vi "STAGE+mono+counter_edit4.vi"() -> ()   [LabVIEW 2017]
panel:
  out "XY Graph":cluster{"Y":dbl[], "Y":dbl[]}[](graph)
  in  "Integrating time, 10^-7 sec":dbl=10000000.0
  out "Timeout 2":bool
  in  "scan from":i32=2600
  in  "scan to":i32=4000
  in  "?":bool
  in  "Exit Labview":bool
  in  "step size":dbl=10.0 min=0.0
  in  "?":bool
  out "Spectrum":waveform(dbl)(graph)
  out "Counts":i32
  in  "value (0)":dbl=-9.0
  out "Current WL Wavelength  2":u16 caption="Current Wavelength"
  out "Grt# 2":u8=1 min=1 max=3 step=1
  out "Blaze (nm)":u32=300
  out "Groove/mm":u32=1200
  in  "?":bool
  in  "Channel B Input":u16(ring)=2 items=["Input 1"=1, "Input 2"=2]
  in  "Trigger mode":u16(ring) items=["10 MHz"=0, "Input 2"=2, "Input T"=3]
  out "Current WL Wavelength":u16 caption="Current Wavelength"
  in  "Integrating time, 10^-7 sec":dbl=10000000.0
  in  "gate A mode (CW:0)":i16(slide) scale=0.0..2.0 scale format="%.2f"
  in  "Channel A Input":u16(ring)=1 items=["10 MHz", "Input 1"]
  in  "Time between measurements\n at one point (s)/Dwell Time":dbl=0.002 min=0.002 max=60.0 step=0.001
  in  "Number of Measurements\n to take at one point/ Number of Periods":u16=1 min=1 max=2000 step=1
  in  "Count Mode":u16(ring) items=["A,B for Preset T", "A-B for Preset T", "A+B for Preset T", "A for Preset B"]
  in  "GPIB address":string="23"
  out "Timeout":bool
  out "Serial":u32=12345
  out "Grt#":u8=1 min=1 max=3 step=1
  out "Blaze (nm)":u32=300
  out "Groove/mm":u32=1200
  out "time delay":u32=450000 min=1
  out "Mono port":T1(ring)
  in  "Get position":bool
  out "Position status":dbl format="%.3f"
  in  "Target position":dbl format="%.3f"
  in  "Move":bool
  in  "Motor OFF":bool
  in  "Motor ON":bool
  in  "Step Size [um]":i32=10
  in  "Axis":i32=1
  in  "Rep Rate [Hz]":dbl=500.0
  out "Shots":dbl
  in  "Averaging Time [s]":dbl=0.1
  out "Current Point":i32
  out "Slide":i32(slide) scale=0.0..100.0
  out "Current Position [mm]":dbl
  in  "Axis initial position [mm]":dbl
  out "Axis final Position [mm]":dbl
  in  "Data Points (100 default)":i32=100
  in  "Collect Data!":bool
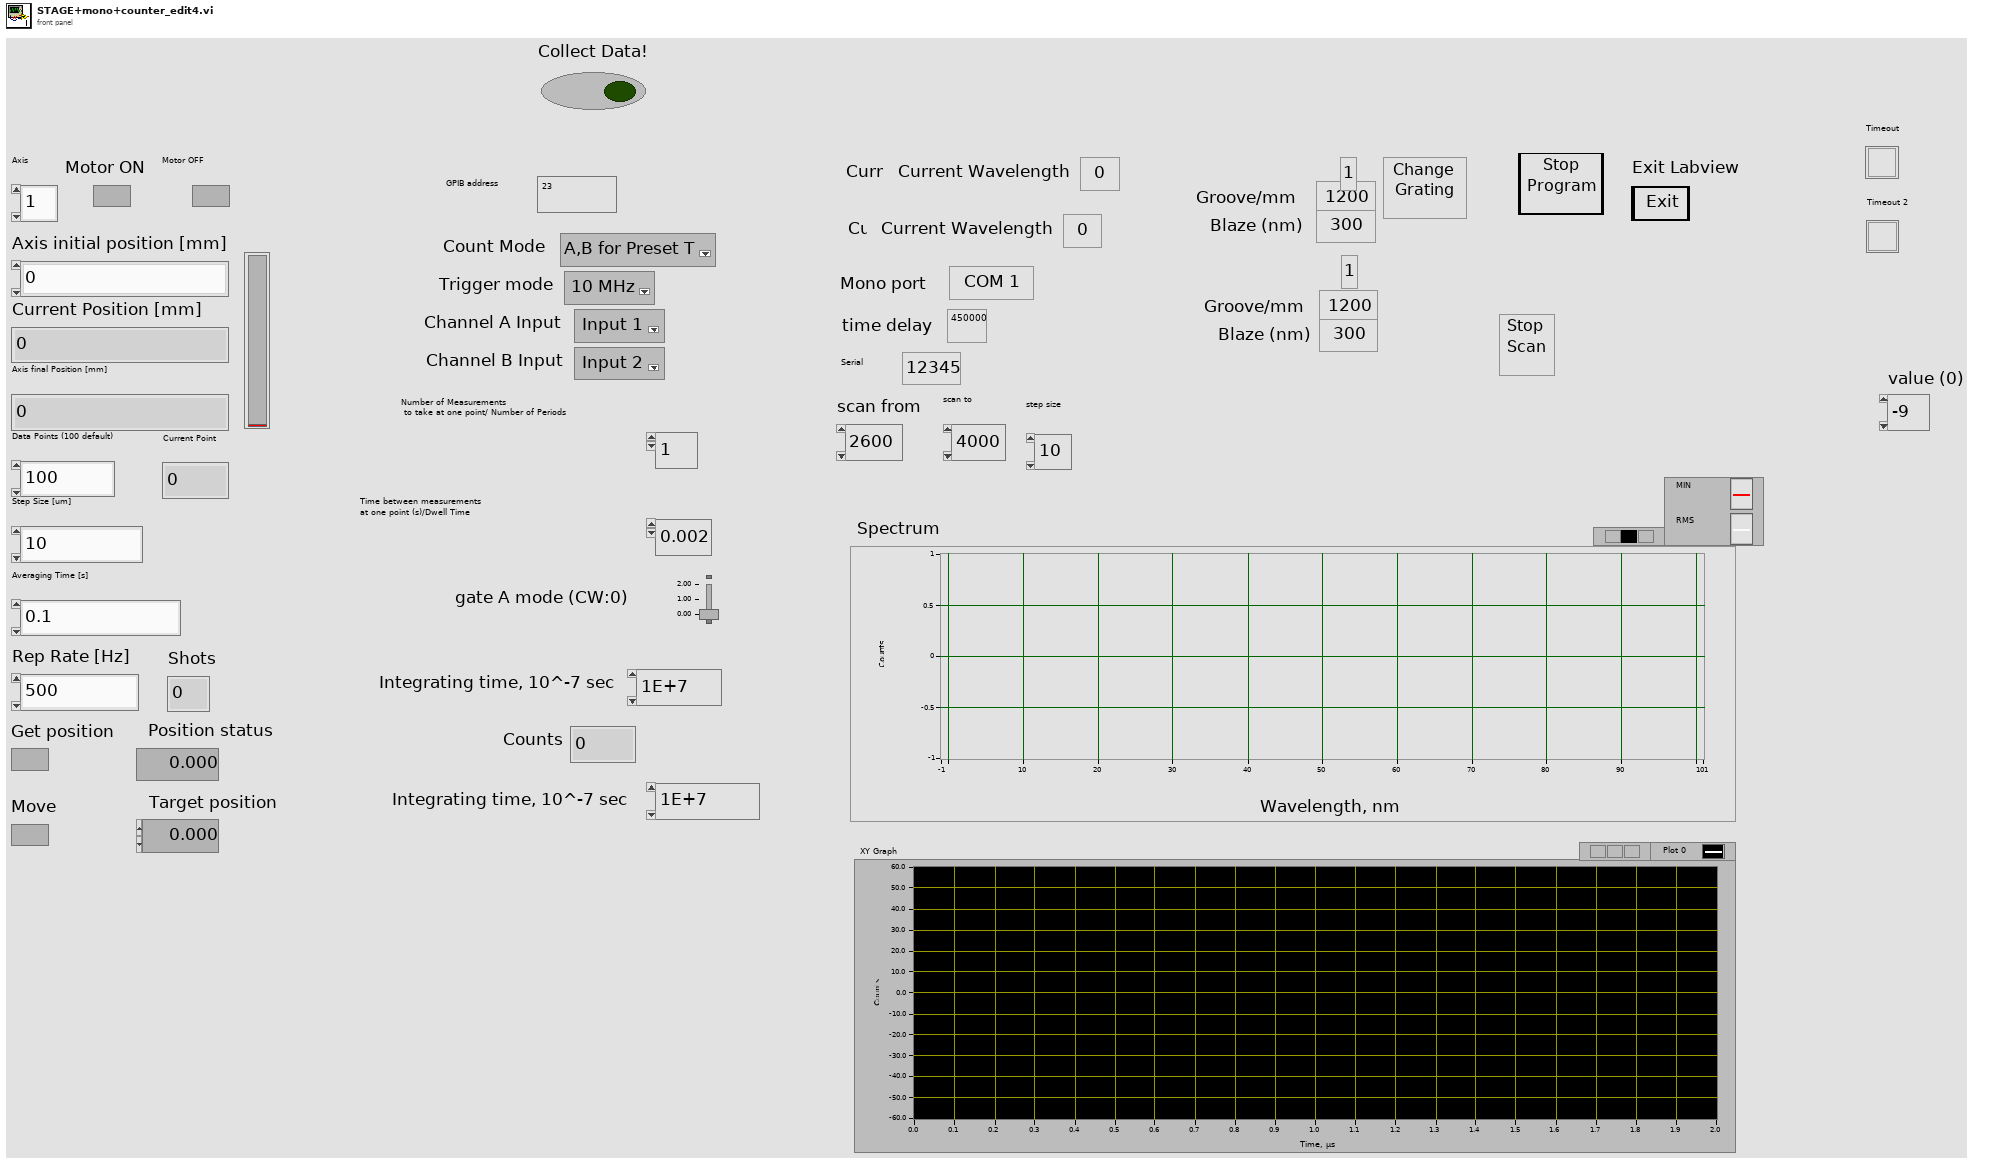
[diagram p1: front panel]
types:
  T1 = enum8{"COM 1", "COM 2", "COM 3", "COM 4", "COM 5", "COM 6", "COM 7", "COM 8", "COM 9"}
  T2 = cluster{"input XON/XOFF":bool, "input HW Handshake":bool, "input alt HW HShk":bool, "output XON/XOFF":bool, "output HW Handshake":bool, "output alt HW HShk":bool, "XOFF byte":u8, "XON byte":u8, "parity error byte":u16}
  T3 = enum16{"no parity", "odd parity", "even parity", "mark parity", "space parity"}
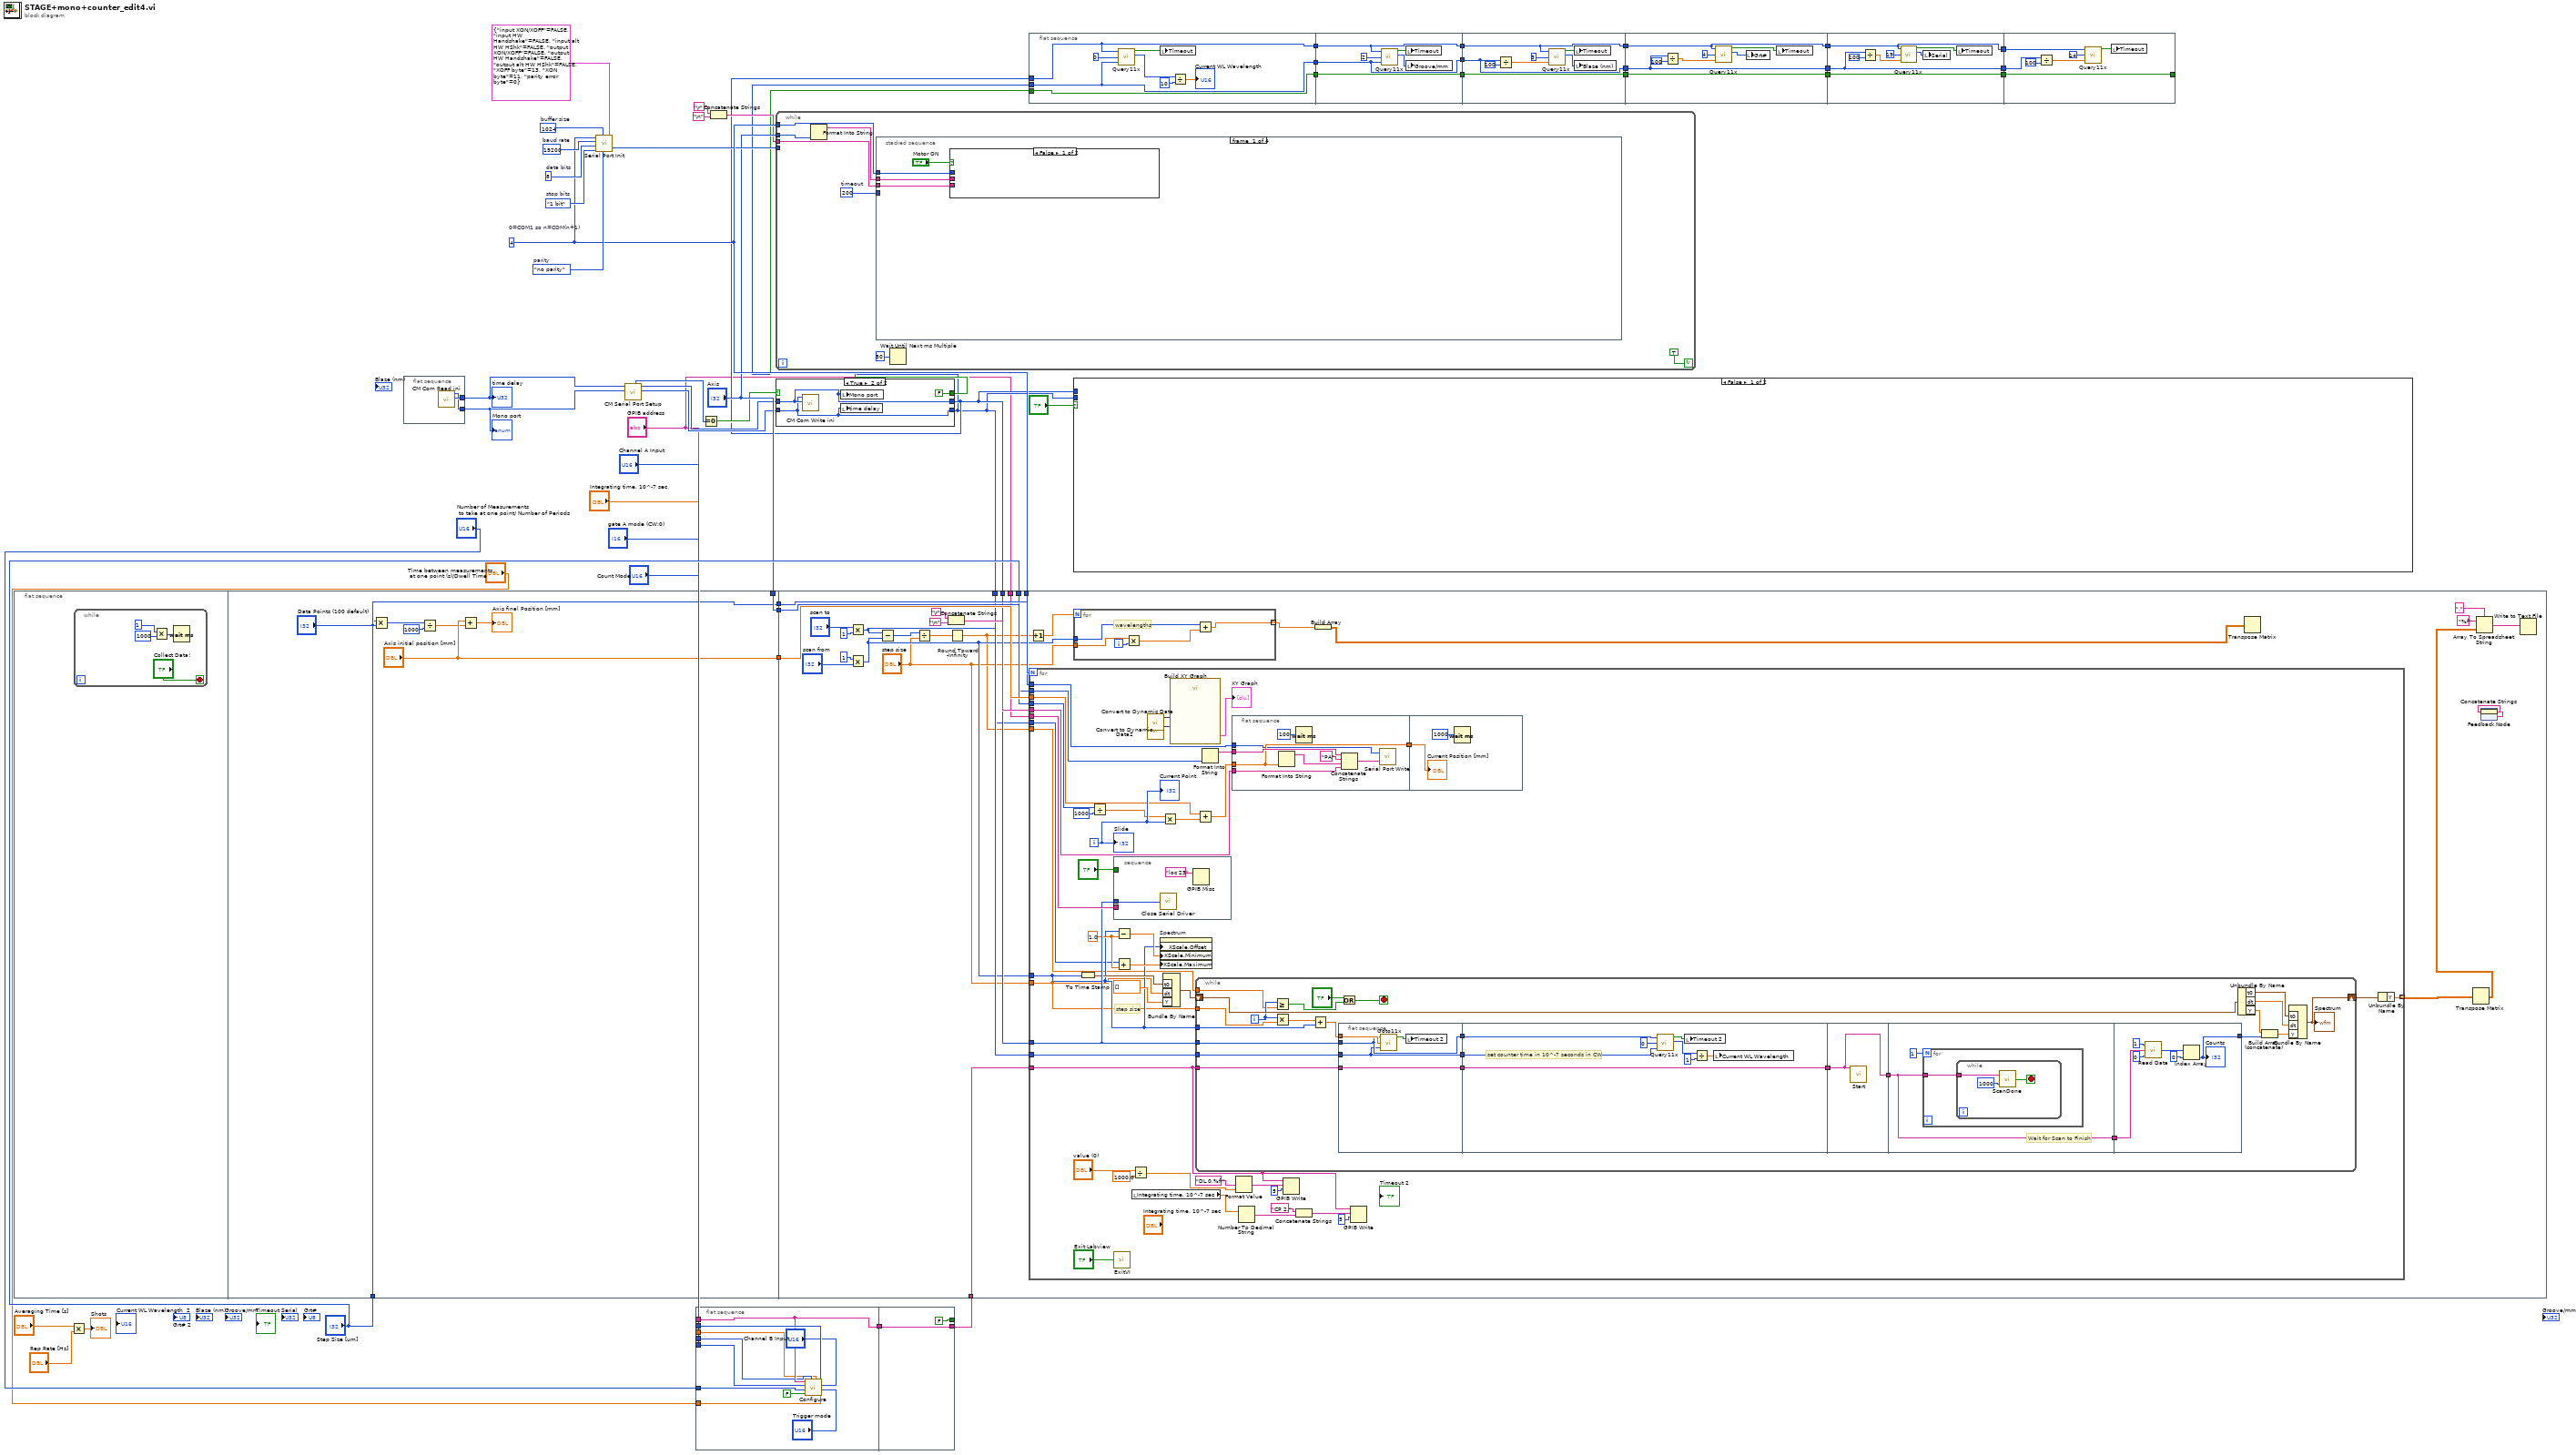
[diagram p0: block diagram]
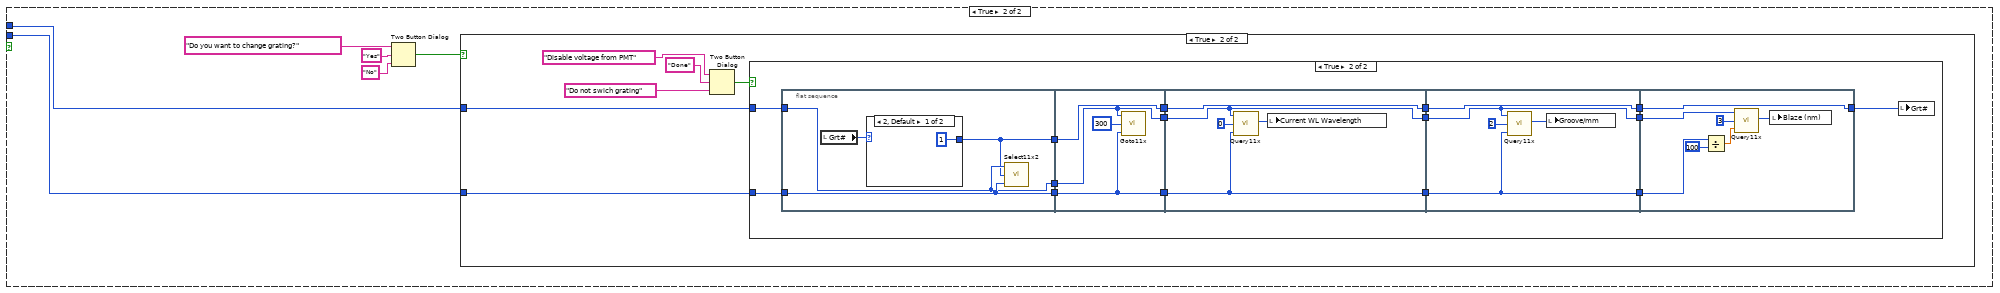
[diagram p2: hidden frame]
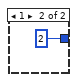
[diagram p5: hidden frame]
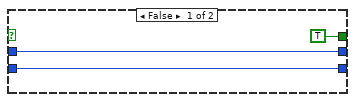
[diagram p6: hidden frame]
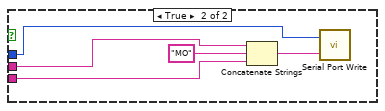
[diagram p7: hidden frame]
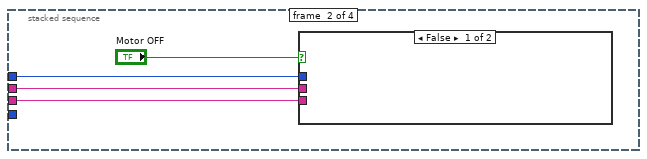
[diagram p8: hidden frame]
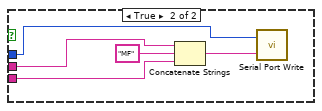
[diagram p9: hidden frame]
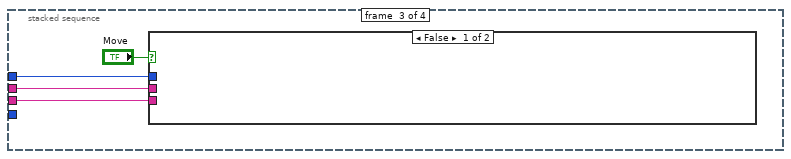
[diagram p10: hidden frame]
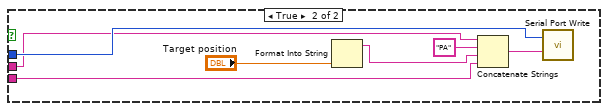
[diagram p11: hidden frame]
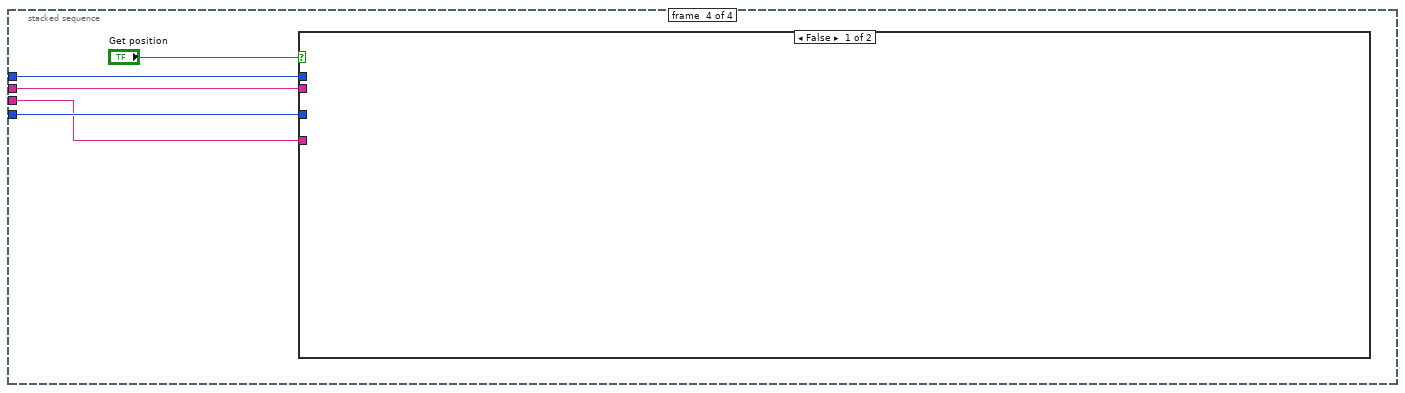
[diagram p12: hidden frame]
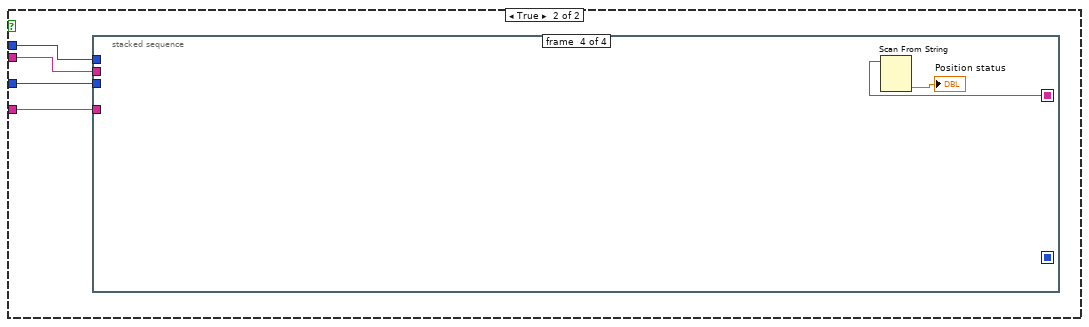
[diagram p13: hidden frame]
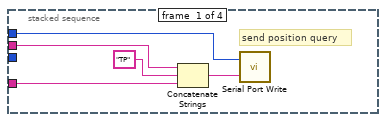
[diagram p14: hidden frame]
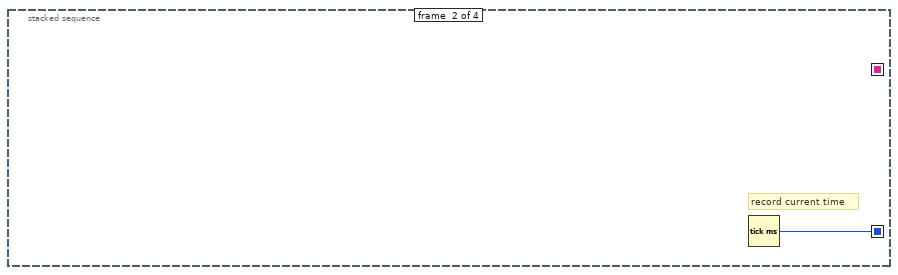
[diagram p15: hidden frame]
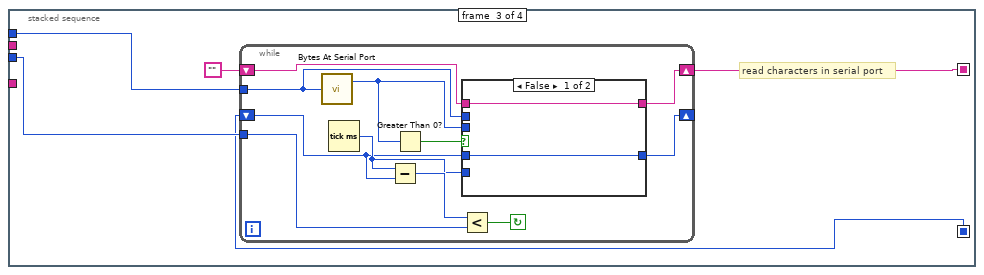
[diagram p16: hidden frame]
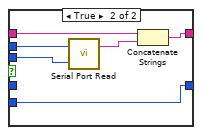
[diagram p17: hidden frame]
diagram:
  w43 = u32 19200  # baud rate
  w42 = u16 8  # data bits
  w41 = enum16{"1 bit", "1.5 bits", "2 bits"}."1 bit"  # stop bits
  w46 = T3."no parity"  # parity
  w40 = 4  # 0=COM1 so n=COM(n+1)
  w45 = u16 1024  # buffer size
  n1 = flat-sequence {
    tunnel: ["Data Points (100 default)"] -> w53
    tunnel: "Axis" -> [w65]
    tunnel: ["Axis initial position [mm]"] -> w52
    tunnel: "Step Size [um]" -> [w58]
    tunnel: [w65] -> w51
    tunnel: w53 -> [w97]
    tunnel: w52 -> [w96]
    tunnel: "Step Size [um]" -> [w95]
    tunnel: w51 -> [w94]
    tunnel: w40 -> [w90]
    tunnel: w4 -> [w89]
    tunnel: w3 -> [w88]
    tunnel: w2 -> [w87]
    tunnel: "GPIB address" -> [w86]
    frame #0 {
      n2 = while {
        stop <- "Collect Data!" stop-if-true
        n3 = Multiply(x=1, y=1000) -> (x*y=w57:i32)
        n4 = Wait (ms)(milliseconds to wait=w57) -> ()  [unwired: 1 out]
      }
    }
    frame #1 {
      n5 = Multiply(x=w58, y="Data Points (100 default)") -> (x*y=w61:i32)
      n6 = Divide(x=w61, y=1000) -> (x/y=w60:dbl)
      n7 = Add(x="Axis initial position [mm]", y=w60) -> (x+y=→"Axis final Position [mm]":dbl)
    }
    frame #2 {
      n8 = Multiply(x="scan to", y=1) -> (x*y=w78:i32)
      n9 = Multiply(x=1, y="scan from") -> (x*y=w81:i32)
      n10 = Subtract(x=w78, y=w81) -> (x-y=w76:i32)
      n11 = Divide(x=w76, y="step size") -> (x/y=w75:dbl)
      n12 = Concatenate Strings("\r", "\n") -> (w91:string)
      n13 = Round Toward -Infinity(1:w75) -> (0:w74:dbl)
      n14 = for {
        N: w97 -> [_]
        tunnel: w96 -> [w145]
        tunnel: w95 -> [w141]
        tunnel: w94 -> [w138]
        tunnel: w91 -> [w135]
        tunnel: w90 -> [w136]
        tunnel: w89 -> [w133]
        tunnel: w88 -> [w130]
        tunnel: w87 -> [w132]
        tunnel: w86 -> [w131]
        tunnel: [w103] -> w67 mode=indexing
        tunnel: w81 -> [w107]
        tunnel: w78 -> [w106]
        tunnel: "step size" -> [w105]
        tunnel: w74 -> [w104]
        i -> [w146]
        w127 = 1.0 ("x")
        # "step size"
        n15 = To Time Stamp(1:w107) -> (0:w123:timestamp)
        n16 = Divide(x=w141, y=1000) -> (x/y=w140:dbl)
        n17 = stacked-sequence {
          tunnel: "?" -> [_]
          tunnel: w130 -> [w199]
          tunnel: w131 -> [_]
          frame #0 {
            n18 = call <vilib>:"Close Serial Driver.vi"("port number"=w199) -> ()  [unwired: 1 out]
            n19 = GPIB Misc(0:"loc 23" ("command string")) -> ()  [unwired: 1 in, 3 out]
          }
        }
        n20 = call "ExitVI.vi"("Exit Labview"="Exit Labview") -> ()
        n21 = Subtract(x=w107, y=w127) -> (x-y=w126:dbl)
        n22 = Add(x=w106, y=w127) -> (x+y=w128:dbl)
        n23 = local read "Integrating time, 10^-7 sec"() -> (w125:dbl)
        n24 = Divide(x="value (0)", y=1000.0) -> (x/y=w111:dbl)
        n25 = call "Convert to Dynamic Data"() -> ("Dynamic Data Type"=w108:dynamicdata)  [unwired: 4 in]
        n26 = call "Convert to Dynamic Data2"() -> ("Dynamic Data Type"=w109:dynamicdata)  [unwired: 4 in]
        n27 = property on="Spectrum" class="WFGraph (strict)"("XScale.Offset"=w107, "XScale.Minimum"=w126, "XScale.Maximum"=w128) -> ()  [unwired: 2 in, 2 out]
        n28 = Multiply(x=w140, y=w146) -> (x*y=w144:dbl)
        n29 = Bundle By Name("t0"=w123, "dt"=w105, "Y"=dbl[] []) -> (w122:waveform(dbl))  [unwired: 1 in]
        n30 = call "Build XY Graph"("Y Input"=w109, "X Input"=w108) -> ("XY Graph"=→"XY Graph":cluster{"Y":dbl[], "Y":dbl[]}[])  [unwired: 3 in, 6 out]
        n31 = while {
          tunnel: w130 -> [w170]
          tunnel: w132 -> [w169]
          shift-right: [w159] -> w117
          shift-left: w122 -> [w167]
          tunnel: w133 -> [w158]
          tunnel: w107 -> [w149]
          tunnel: w105 -> [w148]
          tunnel: w104 -> [w147]
          i -> [w164]
          stop <- w168 stop-if-true
          n32 = Greater Or Equal?(x=w164, y=w147) -> (x >= y?=w160:bool)
          n33 = Multiply(x=w164, y=w148) -> (x*y=w171:dbl)
          n34 = Add(x=w171, y=w149) -> (x+y=w150:dbl)
          n35 = flat-sequence {
            tunnel: w150 -> [w176]
            tunnel: w170 -> [w175]
            tunnel: [w175] -> w156
            tunnel: w169 -> [w174]
            tunnel: [w174] -> w155
            tunnel: w158 -> [w172]
            tunnel: [w172] -> w154
            tunnel: w156 -> [w183]
            tunnel: w155 -> [w182]
            tunnel: w154 -> [w180]
            tunnel: [w180] -> w153
            tunnel: w153 -> [w185]
            tunnel: [w185] -> w152
            tunnel: w152 -> [w186]
            tunnel: [w186] -> w151
            tunnel: w151 -> [w193]
            tunnel: [w192] -> w157
            frame #0 {
              n36 = call "Goto11x.vi"("time delay"=w174, "WAVELENGTH"=w176, "port number"=w175) -> ("timeout"=w173:bool)  [unwired: 2 out]
              n37 = local write "Timeout 2"(w173) -> ()
            }
            frame #1 {
              # "set counter time in 10^-7 seconds in CW"
              n38 = call "Query11x.vi"("port number"=w183, "QUERY"=0, "time delay"=w182) -> ("timeout"=w181:bool, "STATUS MESSAGE"=w179:u16)  [unwired: 2 out]
              n39 = local write "Timeout 2"(w181) -> ()
              n40 = Divide(x=w179, y=1) -> (x/y=w178:dbl)
              n41 = local write "Current WL Wavelength"(w178) -> ()
            }
            frame #2 {
              n42 = call "Start.vi"("GPIB Address"=w185) -> ()  [unwired: 9 in]
            }
            frame #3 {
              # "Wait for Scan to Finish"
              n43 = for {
                N: 1 -> [_]
                tunnel: w186 -> [w188]
                n44 = while {
                  tunnel: w188 -> [w189]
                  stop <- w191 stop-if-true
                  n45 = call "ScanDone.vi"("Wait (ms)"=1000, "GPIB Address"=w189) -> ("Scan Finished?"=w191:bool)
                }
              }
            }
            frame #4 {
              n46 = call "Read Data.vi"("Channel Number"=0, "GPIB Address"=w193, "Number of Datapoints"=1) -> ("Data"=w194:i32[])
              n47 = Index Array(array=w194, index=0) -> (element=w192:i32)
              "Counts" <- w192
            }
          }
          n48 = Or(x="?", y=w160) -> (x .or. y?=w168:bool)
          n49 = Unbundle By Name(w167) -> ("t0"=w165:timestamp, "dt"=w166:dbl, "Y"=w163:dbl[])
          n50 = Build Array (concatenate)(w163, w157) -> (w162:dbl[])
          n51 = Bundle By Name("t0"=w165, "dt"=w166, "Y"=w162) -> (w159:waveform(dbl))  [unwired: 1 in]
          "Spectrum" <- w159
        }
        n52 = Add(x=w145, y=w144) -> (x+y=w143:dbl)
        n53 = Format Into String(w138) -> (resulting string=w137:string)  [unwired: 3 in, 1 out]
        n54 = flat-sequence {
          tunnel: w143 -> [w202]
          tunnel: [w202] -> w139
          tunnel: w135 -> [w204]
          tunnel: w137 -> [w203]
          tunnel: w136 -> [w200]
          tunnel: w139 -> [w208]
          frame #0 {
            n55 = Format Into String(w202) -> (resulting string=w201:string)  [unwired: 3 in, 1 out]
            n56 = Wait (ms)(milliseconds to wait=u32 100) -> ()  [unwired: 1 out]
            n57 = Concatenate Strings(w203, "PA" ("Substring"), w201, w204) -> (w206:string)
            n58 = call <vilib>:"Serial Port Write.vi"("string to write"=w206, "port number"=w200) -> ()  [unwired: 1 out]
          }
          frame #1 {
            n59 = Wait (ms)(milliseconds to wait=u32 1000) -> ()  [unwired: 1 out]
            "Current Position [mm]" <- w208
          }
        }
        n60 = Format Value(format string="DL 0,%f;", value (0)=w111) -> (output string=w115:string)  [unwired: 1 in]
        n61 = Number To Decimal String(number=w125) -> (decimal integer string=w120:string)  [unwired: 1 in]
        n62 = GPIB Write(0:w133, 1:w115, 2:i16 5 ("mode (0)")) -> ()  [unwired: 2 in, 2 out]
        n63 = Concatenate Strings("CP 2,", w120) -> (w118:string)
        n64 = GPIB Write(0:w133, 1:w118, 2:i16 5 ("mode (0)")) -> ()  [unwired: 2 in, 2 out]
        n65 = Unbundle By Name(w117) -> ("Y"=w103:dbl[])
        "Current Point" <- w146
        "Slide" <- w146
      }
      n66 = Increment(x=w74) -> (x+1=w73:dbl)
      n67 = for {
        N: w73 -> [_]
        tunnel: "step size" -> [w102]
        tunnel: w81 -> [w100]
        tunnel: [w98] -> w71 mode=indexing
        i -> [w101]
        # "wavelengths"
        n68 = Multiply(x=w102, y=w101) -> (x*y=w99:dbl)
        n69 = Add(x=w100, y=w99) -> (x+y=w98:dbl)
      }
      n70 = Build Array(w71) -> (w68:dbl[][])
      n71 = Transpose Matrix(1:w68) -> ()  [unwired: 1 out]
      n72 = Transpose Matrix(1:w67) -> (0:w66:dbl[][])
      n73 = Array To Spreadsheet String(delimiter (Tab)=",", array=w66, 3:"%f" ("format string")) -> (spreadsheet string=w72:string)
      n74 = feedback #1() -> (w69:string)  [unwired: 1 in]
      n75 = Concatenate Strings(w69) -> (w70:string)
      n76 = feedback-in #1(w70) -> ()
      n77 = Write to Text File(text=w72) -> ()  [unwired: 3 in, 3 out]
    }
  }
  n78 = Multiply(x="Averaging Time [s]", y="Rep Rate [Hz]") -> (x*y=→"Shots":dbl)
  n79 = flat-sequence {
    tunnel: [w211] -> w18
    tunnel: [w210] -> w17
    frame #0 {
      n80 = call "CM Com Read ini.vi"() -> ("Mono port"=w210:T1, "time delay1"=w211:u32)  [unwired: 7 in]
    }
  }
  n81 = call <vilib>:"Serial Port Init.vi"("flow control etc."=T2 {"input XON/XOFF"=FALSE, "input HW Handshake"=FALSE, "input alt HW HShk"=FALSE, "output XON/XOFF"=FALSE, "output HW Handshake"=FALSE, "output alt HW HShk"=FALSE, "XOFF byte"=13, "XON byte"=11, "parity error byte"=0}, "parity"=w46, "buffer size"=w45, "stop bits"=w41, "data bits"=w42, "baud rate"=w43, "port number"=w40) -> ("error code"=w39:i32)
  n82 = call "CM Serial Port Setup.vi"("COM port"=w17, "time delay"=w18) -> ("time delay1"=w13:u32, "DK port Out"=w14:T1, "error code"=w16:i32)  [unwired: 7 in]
  n83 = flat-sequence {
    tunnel: "GPIB address" -> [w219]
    tunnel: [w219] -> w19
    tunnel: "Count Mode" -> [w220]
    tunnel: "Number of Measurements\n to take at one point/ Number of Periods" -> [w217]
    tunnel: "Time between measurements\n at one point (s)/Dwell Time" -> [w216]
    tunnel: "Channel A Input" -> [w221]
    tunnel: "gate A mode (CW:0)" -> [w213]
    tunnel: "Integrating time, 10^-7 sec" -> [w212]
    tunnel: w19 -> [w222]
    tunnel: [w222] -> w4
    tunnel: [FALSE] -> _
    frame #0 {
      n84 = call "Configure.vi"("Dwell Time (s)"=w216, "Channel T Input"="Trigger mode", "Channel B Input"="Channel B Input", "Channel A Input"=w221, "Integrating time, 10^-7 sec"=w212, "gate mode (CW:0)"=w213, "Scan End Mode"=FALSE, "Number of Periods"=w217, "Count Mode"=w220, "GPIB Address"=w219) -> ()
    }
    frame #1 {
    }
  }
  n85 = Equal To 0?(x=w16) -> (x = 0?=w15:bool)
  n86 = Concatenate Strings("\r", "\n") -> (w35:string)
  n87 = while {
    tunnel: w40 -> [w226]
    tunnel: w35 -> [w227]
    tunnel: w39 -> [_]
    tunnel: "Axis" -> [w224]
    stop <- TRUE continue-if-true
    w225 = u32 200  # timeout
    n88 = Format Into String(w224) -> (resulting string=w228:string)  [unwired: 3 in, 1 out]
    n89 = stacked-sequence {
      tunnel: w228 -> [w232 w242 w251 w263]
      tunnel: w227 -> [w231 w241 w250 w260]
      tunnel: w226 -> [w233 w243 w252 w262]
      tunnel: w225 -> [_ _ _ w261]
      frame #0 {
        n90 = case shown="False" "Motor ON" {
          tunnel: w233 -> [_ w239]
          tunnel: w232 -> [_ w236]
          tunnel: w231 -> [_ w235]
          frame False {
          }
          frame True {
            n91 = Concatenate Strings(w236, "MO" ("Substring"), w235) -> (w237:string)
            n92 = call <vilib>:"Serial Port Write.vi"("string to write"=w237, "port number"=w239) -> ()  [unwired: 1 out]
          }
        }
      }
      frame #1 {
        n93 = case shown="False" "Motor OFF" {
          tunnel: w243 -> [_ w248]
          tunnel: w242 -> [_ w245]
          tunnel: w241 -> [_ w244]
          frame False {
          }
          frame True {
            n94 = Concatenate Strings(w245, "MF" ("Substring"), w244) -> (w246:string)
            n95 = call <vilib>:"Serial Port Write.vi"("string to write"=w246, "port number"=w248) -> ()  [unwired: 1 out]
          }
        }
      }
      frame #2 {
        n96 = case shown="False" "Move" {
          tunnel: w252 -> [_ w259]
          tunnel: w251 -> [_ w256]
          tunnel: w250 -> [_ w255]
          frame False {
          }
          frame True {
            n97 = Format Into String("Target position") -> (resulting string=w253:string)  [unwired: 3 in, 1 out]
            n98 = Concatenate Strings(w256, "PA" ("Substring"), w253, w255) -> (w257:string)
            n99 = call <vilib>:"Serial Port Write.vi"("string to write"=w257, "port number"=w259) -> ()  [unwired: 1 out]
          }
        }
      }
      frame #3 {
        n100 = case shown="False" "Get position" {
          tunnel: w263 -> [_ w268]
          tunnel: w262 -> [_ w267]
          tunnel: w261 -> [_ w266]
          tunnel: w260 -> [_ w265]
          frame False {
          }
          frame True {
            n101 = stacked-sequence {
              seq-local: [_ w274 _ _] -> [_ _ w276 _]
              seq-local: [_ _ w275 _] -> [_ _ _ w300]
              tunnel: w268 -> [w271 _ _ _]
              tunnel: w267 -> [w270 _ w279 _]
              tunnel: w266 -> [_ _ w277 _]
              tunnel: w265 -> [w269 _ _ _]
              frame #0 {
                # "send position query"
                n102 = Concatenate Strings(w271, "TP" ("Substring"), w269) -> (w272:string)
                n103 = call <vilib>:"Serial Port Write.vi"("string to write"=w272, "port number"=w270) -> ()  [unwired: 1 out]
              }
              frame #1 {
                # "record current time"
                n104 = Tick Count (ms)() -> (millisecond timer value=w274:u32)
              }
              frame #2 {
                # "read characters in serial port"
                n105 = while {
                  shift-left: w276 -> [w280]
                  shift-right: [w281] -> _
                  tunnel: w277 -> [w284]
                  shift-left: "" -> [w287]
                  shift-right: [w286] -> w275
                  tunnel: w279 -> [w288]
                  stop <- w283 continue-if-true
                  n106 = call <vilib>:"Bytes At Serial Port.vi"("port number"=w288) -> ("byte count"=w289:u32)  [unwired: 1 out]
                  n107 = Tick Count (ms)() -> (millisecond timer value=w282:u32)
                  n108 = Subtract(x=w282, y=w280) -> (x-y=w285:u32)
                  n109 = Greater Than 0?(x=w289) -> (x > 0?=w290:bool)
                  n110 = case shown="False" w290 {
                    tunnel: w289 -> [_ w298]
                    tunnel: w288 -> [_ w297]
                    tunnel: w287 -> [w292 w295]
                    tunnel: [w292 w294] -> w286
                    tunnel: [w291 w293] -> w281
                    tunnel: w282 -> [_ w293]
                    tunnel: w280 -> [w291 _]
                    frame False {
                    }
                    frame True {
                      n111 = call <vilib>:"Serial Port Read.vi"("requested byte count"=w298, "port number"=w297) -> ("string read"=w296:string)  [unwired: 1 out]
                      n112 = Concatenate Strings(w295, w296) -> (w294:string)
                    }
                  }
                  n113 = Less?(x=w285, y=w284) -> (x < y?=w283:bool)
                }
              }
              frame #3 {
                n114 = Scan From String(input string=w300) -> (output 1=→"Position status":dbl)  [unwired: 4 in, 3 out]
              }
            }
          }
        }
      }
    }
    n115 = Wait Until Next ms Multiple(millisecond multiple=u32 50) -> ()  [unwired: 1 out]
  }
  n116 = case shown="True" w15 {
    tunnel: w14 -> [w303 w306]
    tunnel: w13 -> [w302 w305]
    tunnel: [w303 w306] -> w3
    tunnel: [w302 w305] -> w2
    tunnel: [TRUE FALSE] -> w12
    frame False {
    }
    frame True {
      n117 = call "CM Com Write ini.vi"("time delay1"=w306, "Mono port"=w305) -> ()  [unwired: 7 in]
      n118 = local write "Mono port"(w306) -> ()
      n119 = local write "time delay"(w305) -> ()
    }
  }
  n120 = flat-sequence {
    tunnel: w2 -> [w312]
    tunnel: [w312] -> w34
    tunnel: w3 -> [w314]
    tunnel: [w314] -> w33
    tunnel: w12 -> [w310]
    tunnel: [w310] -> w32
    tunnel: w34 -> [w317]
    tunnel: [w317] -> w31
    tunnel: w33 -> [w319]
    tunnel: [w319] -> w30
    tunnel: w32 -> [w315]
    tunnel: [w315] -> w29
    tunnel: w31 -> [w327]
    tunnel: [w327] -> w28
    tunnel: w30 -> [w324]
    tunnel: [w324] -> w27
    tunnel: w29 -> [w321]
    tunnel: [w321] -> w26
    tunnel: w28 -> [w335]
    tunnel: [w335] -> w25
    tunnel: w27 -> [w332]
    tunnel: [w332] -> w24
    tunnel: w26 -> [w329]
    tunnel: [w329] -> w23
    tunnel: w25 -> [w343]
    tunnel: [w343] -> w22
    tunnel: w24 -> [w340]
    tunnel: [w340] -> w21
    tunnel: w23 -> [w337]
    tunnel: [w337] -> w20
    tunnel: w22 -> [w350]
    tunnel: w21 -> [w347]
    tunnel: [w345] -> _
    tunnel: w20 -> [w345]
    frame #0 {
      n121 = call "Query11x.vi"("port number"=w314, "QUERY"=u16 0, "time delay"=w312) -> ("timeout"=w311:bool, "STATUS MESSAGE"=w309:u16)  [unwired: 2 out]
      n122 = local write "Timeout"(w311) -> ()
      n123 = Divide(x=w309, y=10 ("Numeric")) -> (x/y=→"Current WL Wavelength":dbl)
    }
    frame #1 {
      n124 = call "Query11x.vi"("port number"=w319, "QUERY"=u16 2, "time delay"=w317) -> ("timeout"=w316:bool, "STATUS MESSAGE"=w318:u16)  [unwired: 2 out]
      n125 = local write "Timeout"(w316) -> ()
      n126 = local write "Groove/mm"(w318) -> ()
    }
    frame #2 {
      n127 = Divide(x=w327, y=i16 100 ("device (1)")) -> (x/y=w325:dbl)
      n128 = call "Query11x.vi"("port number"=w324, "QUERY"=u16 3, "time delay"=w325) -> ("timeout"=w322:bool, "STATUS MESSAGE"=w323:u16)  [unwired: 2 out]
      n129 = local write "Timeout"(w322) -> ()
      n130 = local write "Blaze (nm)"(w323) -> ()
    }
    frame #3 {
      n131 = Divide(x=w335, y=i16 100 ("device (1)")) -> (x/y=w333:dbl)
      n132 = call "Query11x.vi"("port number"=w332, "QUERY"=u16 4, "time delay"=w333) -> ("timeout"=w330:bool, "STATUS MESSAGE"=w331:u16)  [unwired: 2 out]
      n133 = local write "Grt#"(w331) -> ()
      n134 = local write "Timeout"(w330) -> ()
    }
    frame #4 {
      n135 = Divide(x=w343, y=i16 100 ("device (1)")) -> (x/y=w341:dbl)
      n136 = call "Query11x.vi"("port number"=w340, "QUERY"=u16 19, "time delay"=w341) -> ("timeout"=w338:bool, "STATUS MESSAGE"=w339:u16)  [unwired: 2 out]
      n137 = local write "Serial"(w339) -> ()
      n138 = local write "Timeout"(w338) -> ()
    }
    frame #5 {
      n139 = Divide(x=w350, y=i16 100 ("device (1)")) -> (x/y=w348:dbl)
      n140 = call "Query11x.vi"("port number"=w347, "QUERY"=u16 14, "time delay"=w348) -> ("timeout"=w346:bool)  [unwired: 3 out]
      n141 = local write "Timeout"(w346) -> ()
    }
  }
  n142 = case shown="False" "?" {
    tunnel: w2 -> [_ w353]
    tunnel: w3 -> [_ w352]
    frame False {
    }
    frame True {
      n143 = Two Button Dialog(message="Do you want to change grating?", 1:"No" ("F button name (\"Cancel\")"), 2:"Yes" ("T button name (\"OK\")")) -> (T button?=w354:bool)
      n144 = case shown="True" w354 {
        tunnel: w353 -> [_ w359]
        tunnel: w352 -> [_ w358]
        frame False {
        }
        frame True {
          n145 = Two Button Dialog(message="Disable voltage from PMT", 1:"Do not swich grating" ("F button name (\"Cancel\")"), 2:"Done" ("T button name (\"OK\")")) -> (T button?=w360:bool)
          n146 = case shown="True" w360 {
            tunnel: w359 -> [_ w378]
            tunnel: w358 -> [_ w377]
            frame False {
            }
            frame True {
              n147 = flat-sequence {
                tunnel: w378 -> [w382]
                tunnel: [w382] -> w375
                tunnel: w377 -> [w381]
                tunnel: [w381] -> w374
                tunnel: [w379] -> w373
                tunnel: w375 -> [w386]
                tunnel: [w386] -> w372
                tunnel: w374 -> [w387]
                tunnel: [w387] -> w371
                tunnel: w373 -> [w385]
                tunnel: [w385] -> w370
                tunnel: w372 -> [w393]
                tunnel: [w393] -> w369
                tunnel: w371 -> [w392]
                tunnel: [w392] -> w368
                tunnel: w370 -> [w389]
                tunnel: [w389] -> w367
                tunnel: w369 -> [w396]
                tunnel: [w396] -> w366
                tunnel: w368 -> [w397]
                tunnel: [w397] -> w365
                tunnel: w367 -> [w394]
                tunnel: [w394] -> w364
                tunnel: w366 -> [w401]
                tunnel: w365 -> [w402]
                tunnel: [w399] -> w376
                tunnel: w364 -> [w399]
                frame #0 {
                  n148 = local read "Grt#"() -> (w380:u8)
                  n149 = case shown="2, Default" w380 {
                    tunnel: [1 2] -> w379
                    frame 2, Default {
                    }
                    frame 1 {
                    }
                  }
                  n150 = call "Select11x2.vi"("time delay"=w382, "NEW GRT?"=w379, "port number"=w381) -> ()  [unwired: 3 out]
                }
                frame #1 {
                  n151 = call "Goto11x.vi"("time delay"=w386, "WAVELENGTH"=u16 300, "port number"=w387) -> ()  [unwired: 3 out]
                }
                frame #2 {
                  n152 = call "Query11x.vi"("port number"=w392, "QUERY"=u16 0, "time delay"=w393) -> ("STATUS MESSAGE"=w390:u16)  [unwired: 3 out]
                  n153 = local write "Current WL Wavelength"(w390) -> ()
                }
                frame #3 {
                  n154 = call "Query11x.vi"("port number"=w397, "QUERY"=u16 2, "time delay"=w396) -> ("STATUS MESSAGE"=w395:u16)  [unwired: 3 out]
                  n155 = local write "Groove/mm"(w395) -> ()
                }
                frame #4 {
                  n156 = Divide(x=w401, y=i16 100 ("device (1)")) -> (x/y=w403:dbl)
                  n157 = call "Query11x.vi"("port number"=w402, "QUERY"=u16 3, "time delay"=w403) -> ("STATUS MESSAGE"=w400:u16)  [unwired: 3 out]
                  n158 = local write "Blaze (nm)"(w400) -> ()
                }
              }
              n159 = local write "Grt#"(w376) -> ()
            }
          }
        }
      }
    }
  }
  "Mono port" <- w17
  "time delay" <- w18
